vi "HRTF-Options Dialog.vi"(0 "Options in":T1) -> (4 "Options out":T1, 8 "Canceled?":bool)   [LabVIEW 2015]
uses:
  Typedefs/HRTF-Options.ctl
panel:
  in  "Wait (s)":dbl caption="Wait between measurements (s)"
  in  "Elevations":string
  in  "Root folder":path
  out "exit signal":bool
  in  "Cancel":bool
  in  "OK":bool
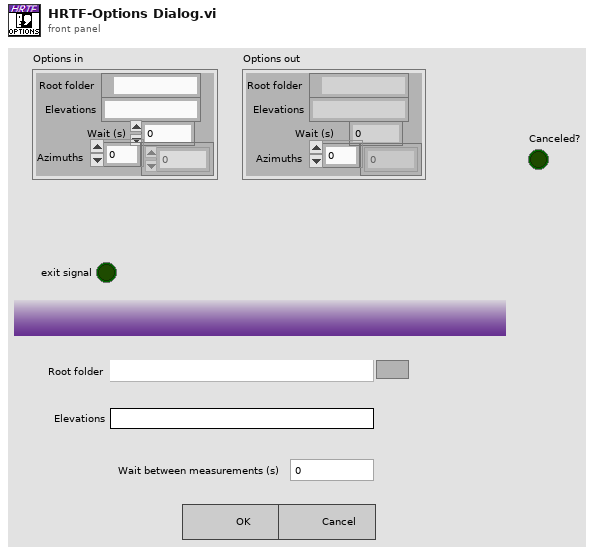
[diagram p1: front panel]
types:
  T1 = typedef "HRTF-Options.ctl" = cluster{"Root folder":path, "Elevations":string, "Wait (s)":dbl, "Azimuths":dbl[]}
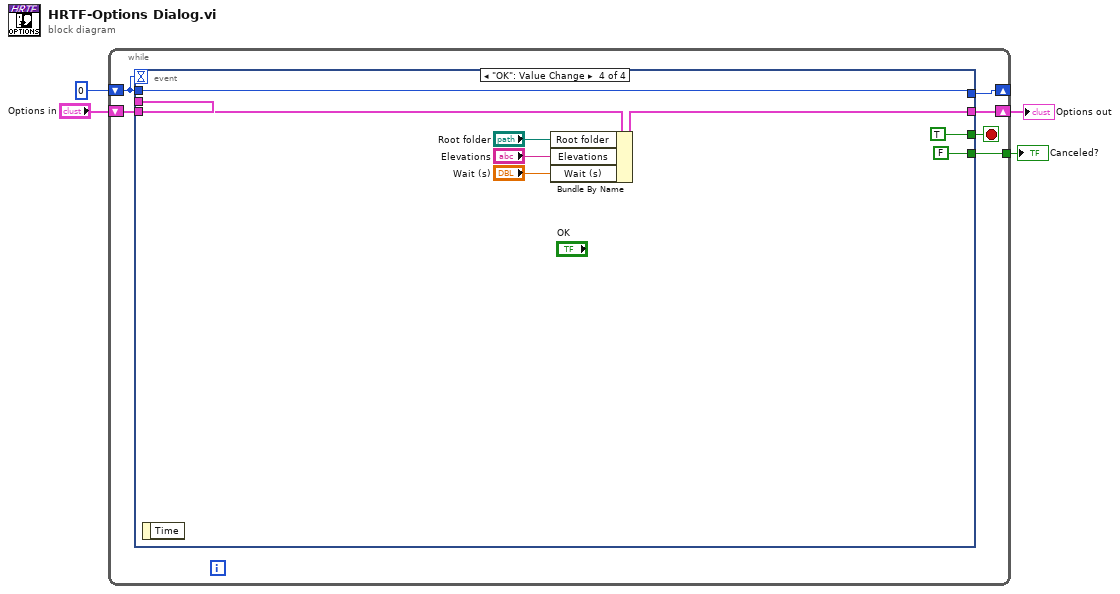
[diagram p0: block diagram]
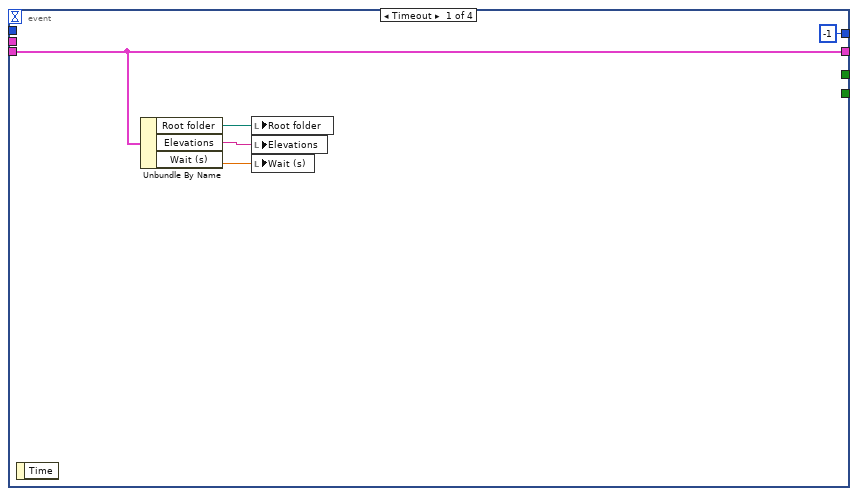
[diagram p2: hidden frame]
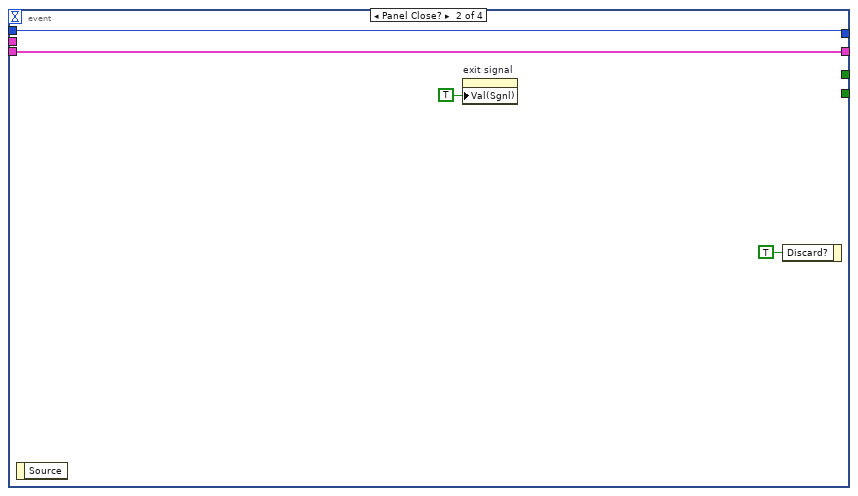
[diagram p3: hidden frame]
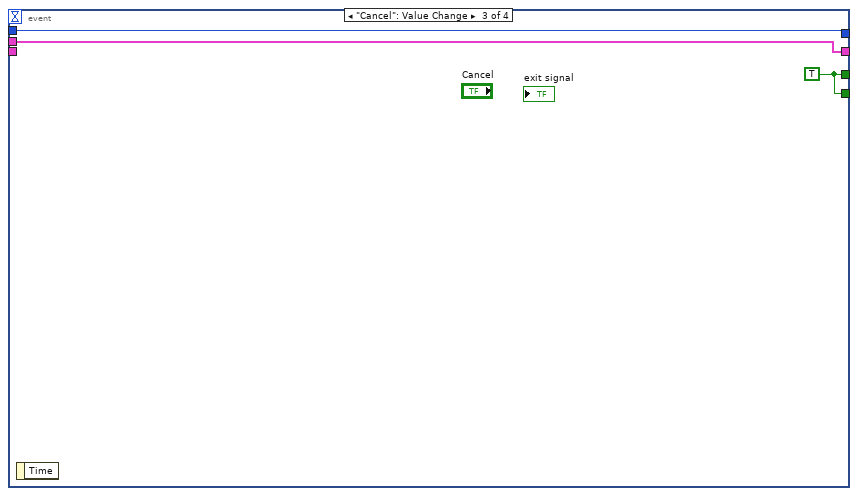
[diagram p4: hidden frame]
diagram:
  n1 = while {
    shift-right: [w10] -> _
    shift-left: 0 -> [w5]
    tunnel: [w7] -> w1
    shift-right: [w9] -> w2
    shift-left: "Options in" -> [w6]
    stop <- w8 stop-if-true
    n2 = event shown="[3] \"OK\": Value Change" {
      selector: _ -> [_ _ _ _]
      dyn-events: _ -> [_ _ _ _]
      timeout: w5 -> [_ _ _ _]
      tunnel: [-1 w19 w20 w27] -> w10
      tunnel: w6 -> [w14 w18 _ w30]
      tunnel: [w14 w18 w21 w26] -> w9
      tunnel: [_ _ w22 TRUE] -> w8
      tunnel: [_ _ w22 FALSE] -> w7
      tunnel: w6 -> [_ _ w21 _]
      tunnel: w5 -> [_ w19 w20 w27]
      event Timeout {
        n3 = event-data() -> ()  [unwired: 1 in, 1 out]
        n4 = Unbundle By Name(w14) -> ("Root folder"=w13:path, "Elevations"=w12:string, "Wait (s)"=w11:dbl)
        n5 = local write "Root folder"(w13) -> ()
        n6 = local write "Elevations"(w12) -> ()
        n7 = local write "Wait (s)"(w11) -> ()
      }
      event Panel Close? {
        n8 = event-data() -> ()  [unwired: 1 in, 1 out]
        n9 = property on="exit signal" class="Bool (strict)"("Val(Sgnl)"=TRUE ("Value (Signaling)")) -> ()  [unwired: 2 in, 2 out]
        n10 = event-data("Discard?"=TRUE) -> ()  [unwired: 1 in, 1 out]
      }
      event "Cancel": Value Change {
        w22 = TRUE
        n11 = event-data() -> ()  [unwired: 1 in, 1 out]
      }
      event "OK": Value Change {
        n12 = event-data() -> ()  [unwired: 1 in, 1 out]
        n13 = Bundle By Name(cluster=w30, "Root folder"="Root folder", "Elevations"="Elevations", "Wait (s)"="Wait (s)") -> (w26:T1)
      }
    }
  }
  "Options out" <- w2
  "Canceled?" <- w1
